vi "Start Module.vi"(8 "error in (no error)":errorcluster) -> (0 "error out":errorcluster, 1 "Wait for Event Sync?":bool, 2 "Server Broadcast Events":T1, 3 "Module Was Already Running?":bool)   [LabVIEW 2015, in "Server.lvlib"]
doc: "Launches the Module Main.vi.\n_____\nBased on Delacor QMH Project Template 4.2.1.64."
uses:
  Server.lvlib
  Broadcast Events--cluster.ctl
  Did Init Argument--cluster.ctl
  Status Updated Argument--cluster.ctl
  Error Reported Argument--cluster.ctl
  Stop Argument--cluster.ctl
  Get Module Execution Status Argument--cluster.ctl
  <vilib>/Delacor/Delacor QMH/Libraries/Module Admin_class/Delacor_lib_QMH_Module Admin.lvclass
  <vilib>/Delacor/Delacor QMH/Libraries/Module Admin_class/Delacor_lib_QMH_Module Admin.lvclass/Delacor_lib_QMH_Module Admin.ctl
  <vilib>/Delacor/Delacor QMH/Libraries/Module Admin_class/Delacor_lib_QMH_Set External Launch.vi
  <vilib>/Utility/error.llb/Error Cluster From Error Code.vi
  <vilib>/ErrorRing/Error Ring.xnode
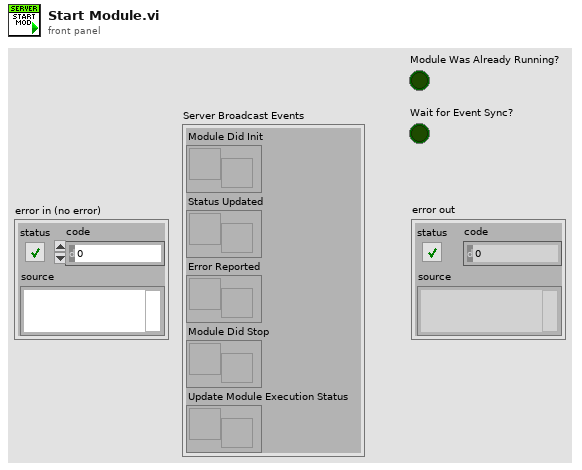
[diagram p1: front panel]
types:
  T1 = typedef "Server.lvlib/Broadcast Events--cluster.ctl" = cluster{"Module Did Init":refnum<user-event>, "Status Updated":refnum<user-event>, "Error Reported":refnum<user-event>, "Module Did Stop":refnum<user-event>, "Update Module Execution Status":refnum<user-event>}
  T2 = enum32{"Bad", "Idle", "Run top level", "Running"}
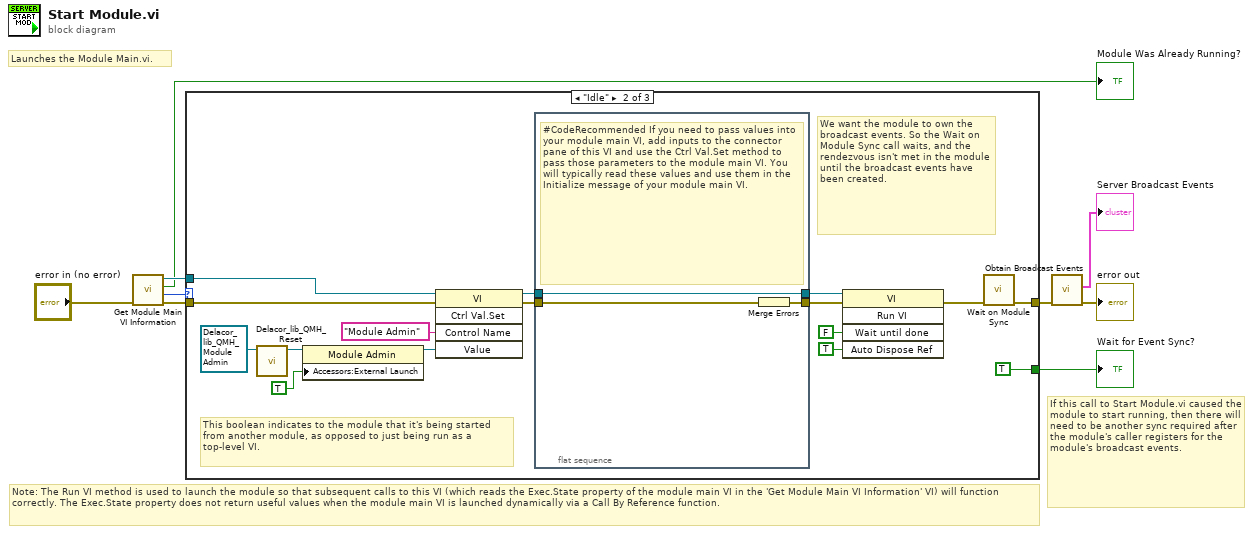
[diagram p0: block diagram]
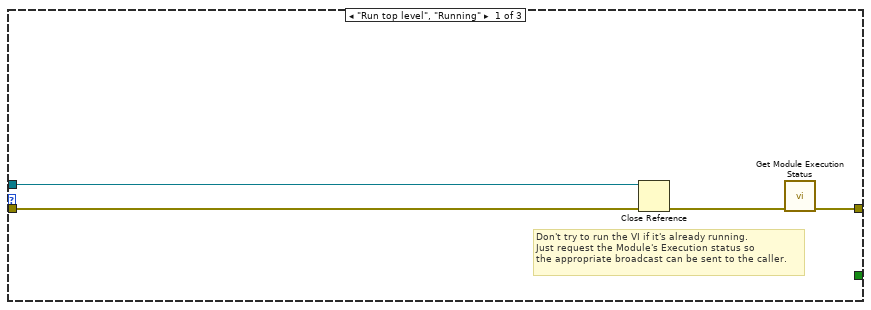
[diagram p2: hidden frame]
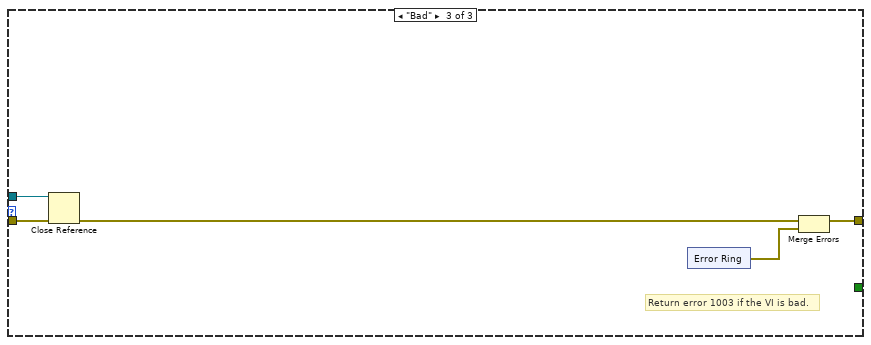
[diagram p3: hidden frame]
diagram:
  # "Note: The Run VI method is used to launch the module so that subsequent calls to this VI (which reads the Exec.State property of the module main VI in the 'Get Module Main VI Information' VI) will function correctly. The Exec.State property does not return useful values when the module main VI is launched dynamically via a Call By Reference function."
  # "If this call to Start Module.vi caused the module to start running, then there will need to be another sync required after the module's caller registers for the module's broadcast events."
  # "Launches the Module Main.vi."
  n1 = call "Get Module Main VI Information.vi"("error in (no error)"="error in (no error)") -> ("error out"=w8:errorcluster, "Execution State"=w3:T2, "Is Module Running?"=→"Module Was Already Running?":bool, "Module Main VI"=w7:refnum<vi>)  [unwired: 7 in]
  n2 = case shown="\"Idle\"" w3 {
    tunnel: w8 -> [w13 w27 w37]
    tunnel: w7 -> [w12 w28 w36]
    tunnel: [w10 w23 w34] -> w6
    tunnel: [_ TRUE _] -> w4
    frame "Run top level", "Running" {
      # "Don't try to run the VI if it's already running.\nJust request the Module's Execution status so\nthe appropriate broadcast can be sent to the caller."
      n3 = Close Reference(reference=w12, error in (no error)=w13) -> (error out=w11:errorcluster)
      n4 = call "Get Module Execution Status.vi"("error in (no error)"=w11) -> ("error out"=w10:errorcluster)  [unwired: 10 in]
    }
    frame "Idle" {
      # "We want the module to own the broadcast events. So the Wait on Module Sync call waits, and the rendezvous isn't met in the module until the broadcast events have been created."
      # "This boolean indicates to the module that it's being started from another module, as opposed to just being run as a top-level VI."
      n5 = call-dynamic "Delacor_lib_QMH_Reset.vi"("Mod Admin in"=refnum<class "Delacor_lib_QMH_Module Admin.lvclass"> refnum) -> ("Mod Admin out"=w21:refnum<class "Delacor_lib_QMH_Module Admin.lvclass">)  [unwired: 9 in, 1 out]
      n6 = property class="Module Admin"(reference=w21, "Accessors:External Launch"=TRUE) -> (reference out=w18:refnum<class "Delacor_lib_QMH_Module Admin.lvclass">)  [unwired: 1 in, 1 out]
      n7 = invoke class="VI" method="Ctrl Val.Set"(reference=w28, error in=w27, "Control Name"="Module Admin", "Value"=w18) -> (reference out=w17:refnum<vi>, error out=w15:errorcluster)  [unwired: 1 in, 3 out]
      n8 = flat-sequence {
        tunnel: w17 -> [w32]
        tunnel: [w32] -> w16
        tunnel: w15 -> [w31]
        tunnel: [w30] -> w14
        frame #0 {
          # "#CodeRecommended If you need to pass values into your module main VI, add inputs to the connector pane of this VI and use the Ctrl Val.Set method to pass those parameters to the module main VI. You will typically read these values and use them in the Initialize message of your module main VI."
          n9 = Merge Errors(w31) -> (w30:errorcluster)
        }
      }
      n10 = invoke class="VI" method="Run VI"(reference=w16, error in=w14, "Wait until done"=FALSE ("Wait Until Done"), "Auto Dispose Ref"=TRUE ("Auto Dispose Reference")) -> (error out=w24:errorcluster)  [unwired: 1 in, 4 out]
      n11 = call "Wait on Module Sync.vi"("error in (no error)"=w24) -> ("error out"=w23:errorcluster)  [unwired: 10 in]
    }
    frame "Bad" {
      # "Return error 1003 if the VI is bad."
      n12 = Close Reference(reference=w36, error in (no error)=w37) -> (error out=w35:errorcluster)
      n13 = xnode "Error Ring"() -> ("error out"=w33:errorcluster)
      n14 = Merge Errors(w35, w33) -> (w34:errorcluster)
    }
  }
  "Wait for Event Sync?" <- w4
  n15 = call "Obtain Broadcast Events.vi"("error in (no error)"=w6) -> ("error out"=→"error out":errorcluster, "Server Broadcast Events"=→"Server Broadcast Events":T1)  [unwired: 9 in]
